vi "Set TreeSettings.vi"(8 "error in (no error)":errorcluster, 10 "TreeSettings":T1, 11 "VariantTree.lvclass in":refnum<class "VariantTree__VP.lvclass">) -> (0 "error out":errorcluster, 3 "VariantTree.lvclass out":refnum<class "VariantTree__VP.lvclass">)   [LabVIEW 2011, in "VariantTree__VP.lvclass"]
uses:
  VariantTree__VP.lvclass
  TreeSettings.ctl
  VariantTree__VP.lvclass/VariantTree__VP.ctl
  VariantXControl__VP.xctl
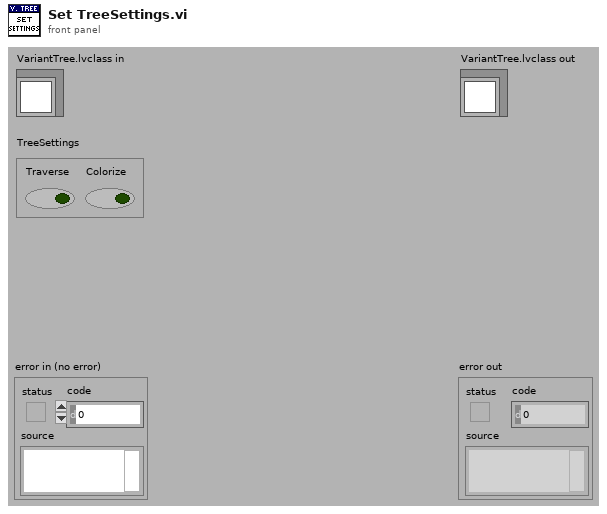
[diagram p1: front panel]
types:
  T1 = typedef "VariantXControl__VP.xctl/TreeSettings.ctl" = cluster{"Traverse":bool, "Colorize":bool}
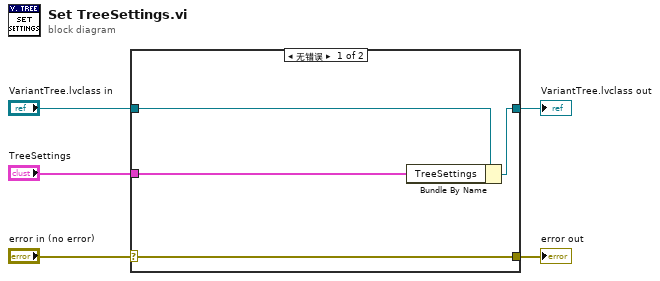
[diagram p0: block diagram]
diagram:
  n1 = case shown="无错误" "error in (no error)" {
    selector: "error in (no error)" -> [w9 w10]
    tunnel: [w9 w10] -> w4
    tunnel: [w7 w11] -> w2
    tunnel: "VariantTree.lvclass in" -> [w8 w11]
    tunnel: "TreeSettings" -> [w6 _]
    frame No Error {
      n2 = Bundle By Name(cluster=w8, "TreeSettings"=w6) -> (w7:refnum<class "VariantTree__VP.lvclass">)
    }
    frame Error {
    }
  }
  "error out" <- w4
  "VariantTree.lvclass out" <- w2
